vi "Encoder_To_Degrees.vi"(8 "Max Encoder Value":dbl=0.51, 9 "Degrees Rotation":dbl=250.0, 11 "Encoder Value":dbl) -> (3 "Degree Value":dbl)   [LabVIEW 2011]
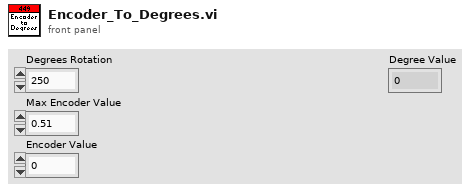
[diagram p1: front panel]
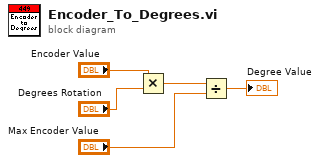
[diagram p0: block diagram]
diagram:
  n1 = Multiply(x="Encoder Value", y="Degrees Rotation") -> (x*y=w5:dbl)
  n2 = Divide(x=w5, y="Max Encoder Value") -> (x/y=→"Degree Value":dbl)
